vi "Check Abort Stop.vi"(8 "error in (no error)":refnum<class "MultiErrors.lvclass">, 11 "Sequence Validation in":refnum<class "Sequence Validation.lvclass">) -> (0 "error out":refnum<class "MultiErrors.lvclass">, 3 "Sequence Validation out":refnum<class "Sequence Validation.lvclass">)   [LabVIEW 2020, in "VolatusSeq.lvlib" / "Sequence Validation.lvclass"]
uses:
  Sequence Validation.lvclass
  Sequence Validation.lvclass/Sequence Validation.ctl
  Sequence Config/Sequence Config.lvclass
  VolatusErrorUtilities/MultiErrors/MultiErrors.lvclass
  Command Type.ctl
  VolatusSeqConfig.lvlib
  Command Config/Command Config.lvclass
  Transition Command Config/Transition Command Config.lvclass
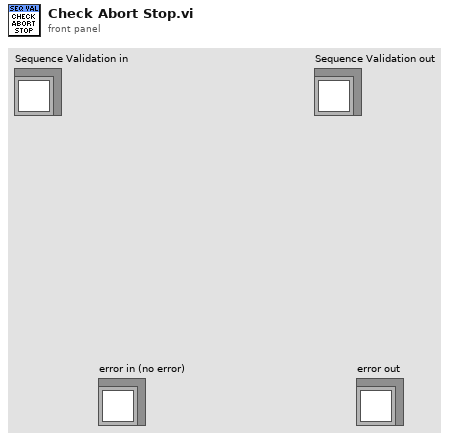
[diagram p1: front panel]
types:
  T1 = typedef "VolatusSeqConfig.lvlib/Command Type.ctl" = enum16{"Digital", "Numeric", "Transition", "Stop", "StartLog", "StopLog", "Start", "Event", "Error", "HTTP", "ResetVar", "IncVar", "DecVar", "SaveVar", "LoadVar", "AddVar", "SubVar", "SetVar"}
  T2 = typedef "VolatusSeqConfig.lvlib/State.ctl" = cluster{"Name":string, "Steps":T3[], "Transitions":refnum<class "Transition Config.lvclass">[], "Comment":string, "Color":string, "Seq Name":string, "Report Conditions":bool}
  T3 = typedef "VolatusSeqConfig.lvlib/Step.ctl" = cluster{"Time":dbl, "Commands":refnum<class "Command Config.lvclass">[]}
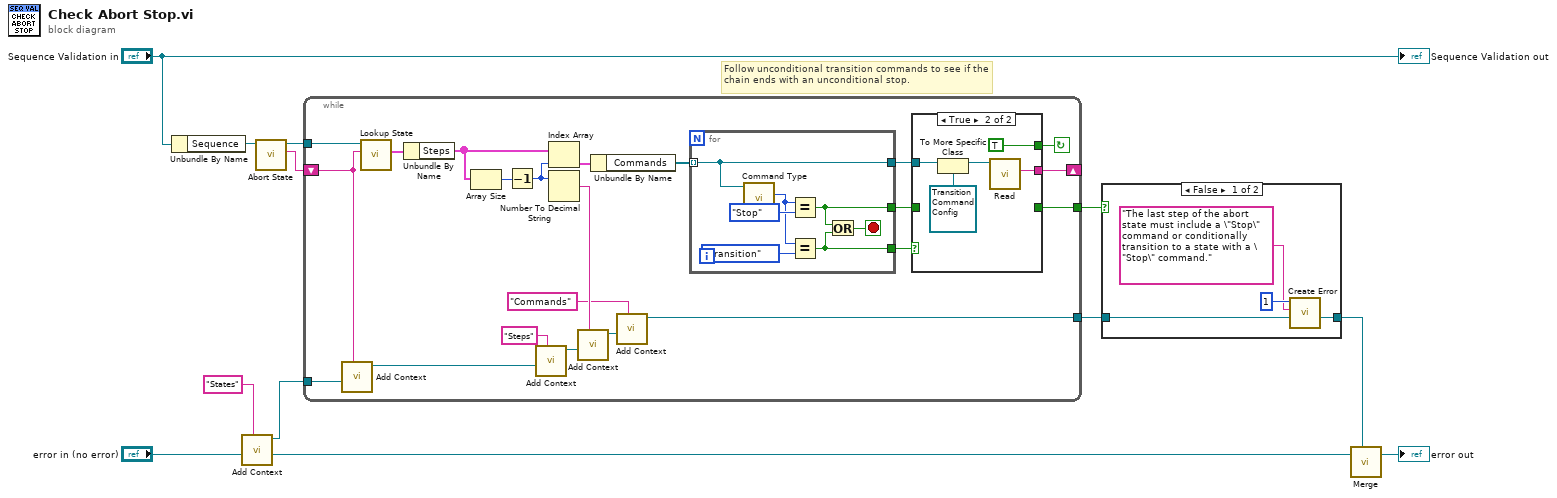
[diagram p0: block diagram]
diagram:
  # "Follow unconditional transition commands to see if the chain ends with an unconditional stop."
  n1 = Unbundle By Name("Sequence Validation in") -> ("Sequence"=w10:refnum<class "Sequence Config.lvclass">)
  n2 = call "Add Context.vi"("Context"="States", "MultiErrors in"="error in (no error)") -> ("Original Context"=w8:refnum<class "MultiErrors.lvclass">, "Added Context"=w6:refnum<class "MultiErrors.lvclass">)  [unwired: 8 in]
  n3 = call "Abort State.vi"("Sequence Config in"=w10) -> ("Abort State"=w5:string, "Sequence Config out"=w9:refnum<class "Sequence Config.lvclass">)  [unwired: 9 in]
  n4 = while {
    tunnel: w9 -> [w34]
    tunnel: [w14] -> w4
    shift-right: [w16] -> _
    shift-left: w5 -> [w31]
    tunnel: w6 -> [w32]
    tunnel: [w19] -> w3
    stop <- w15 continue-if-true
    n5 = call "Add Context.vi"("Context"=w31, "MultiErrors in"=w32) -> ("Added Context"=w30:refnum<class "MultiErrors.lvclass">)  [unwired: 8 in, 1 out]
    n6 = call "Lookup State.vi"("State"=w31, "Sequence Config in"=w34) -> ("Info"=w33:T2)  [unwired: 7 in, 2 out]
    n7 = Unbundle By Name(w33) -> ("Steps"=w27:T3[])
    n8 = Array Size(array=w27) -> (size(s)=w28:i32)
    n9 = Decrement(x=w28) -> (x-1=w24:i32)
    n10 = call "Add Context.vi"("Context"="Steps", "MultiErrors in"=w30) -> ("Added Context"=w25:refnum<class "MultiErrors.lvclass">)  [unwired: 8 in, 1 out]
    n11 = Index Array(array=w27, index=w24) -> (element=w26:T3)
    n12 = Number To Decimal String(number=w24) -> (decimal integer string=w23:string)  [unwired: 1 in]
    n13 = call "Add Context.vi"("Context"=w23, "MultiErrors in"=w25) -> ("Added Context"=w22:refnum<class "MultiErrors.lvclass">)  [unwired: 8 in, 1 out]
    n14 = Unbundle By Name(w26) -> ("Commands"=w20:refnum<class "Command Config.lvclass">[])
    n15 = call "Add Context.vi"("Context"="Commands", "MultiErrors in"=w22) -> ("Added Context"=w19:refnum<class "MultiErrors.lvclass">)  [unwired: 8 in, 1 out]
    n16 = for {
      tunnel: w20 -> [w41] mode=indexing
      tunnel: [w44] -> w13
      tunnel: [w42] -> w18
      tunnel: [w41] -> w17
      stop <- w43 stop-if-true
      n17 = call-dynamic "Command Type.vi"("Command Config in"=w41) -> ("Command Type"=w45:T1)  [unwired: 10 in]
      n18 = Equal?(x=w45, y=Command_Type."Stop") -> (x = y?=w44:bool)
      n19 = Equal?(x=w45, y=Command_Type."Transition") -> (x = y?=w42:bool)
      n20 = Or(x=w44, y=w42) -> (x .or. y?=w43:bool)
    }
    n21 = case shown="True" w18 {
      tunnel: w17 -> [_ w38]
      tunnel: [_ w39] -> w16
      tunnel: [_ TRUE] -> w15
      tunnel: [w35 _] -> w14
      tunnel: w13 -> [w35 _]
      frame False {
      }
      frame True {
        n22 = To More Specific Class(target class=refnum<class "Transition Command Config.lvclass"> refnum ("VolatusSeqConfig.lvlib:Transition Command Config.lvclass"), reference=w38) -> (specific class reference=w36:refnum<class "Transition Command Config.lvclass">)  [unwired: 1 in, 1 out]
        n23 = call "Read.vi"("Transition Command Config in"=w36) -> ("Target"=w39:string)  [unwired: 8 in, 2 out]
      }
    }
  }
  n24 = case shown="False" w4 {
    tunnel: w3 -> [w51 w52]
    tunnel: [w48 w52] -> w1
    frame False {
      n25 = call "Create Error.vi"("MultiErrors in"=w51, "Message"="The last step of the abort state must include a \"Stop\" command or conditionally transition to a state with a \"Stop\" command.", "Code"=1) -> ("MultiErrors out"=w48:refnum<class "MultiErrors.lvclass">)  [unwired: 8 in]
    }
    frame True {
    }
  }
  n26 = call "Merge.vi"("First Error In"=w8, "Second Error In"=w1) -> ("MultiErrors out"=→"error out":refnum<class "MultiErrors.lvclass">)  [unwired: 5 in]
  "Sequence Validation out" <- "Sequence Validation in"
